vi "Upload Firmware.vi"(5 "Progress Bar":refnum<vi>, 6 "AVRDUDE Timeout (45000)":u32=45000, 7 "COM Port":refnum<visa-resource-name>="COM5", 8 "Error In":errorcluster, 9 "Firmware Index":u16(ring) items=["LINX -  Serial / USB", "LINX -  Serial / USB [Debug] "], 10 "Device Index":u16=1, 11 "Family Index":dbl=1.0) -> (0 "Error Out":errorcluster={"status"=TRUE, "code"=-1073807346, "source"="VISA Open in LVH-LINX.lvlib:Upload Firmware.vi"}, 2 "Success?":bool)   [LabVIEW 2011, in "LVH-LINX.lvlib"]
uses:
  LVH-LINX.lvlib
  Type Defs/All Firmware Data FGV States.ctl
  <vilib>/LabVIEW Hacker/LVH-Toolbox/Common/LVH-Common.lvlib
  Type Defs/Devices - Arduino.ctl
  Type Defs/Devices - Digilent.ctl
  Device/Device.lvlib
panel:
  out "Success?":bool
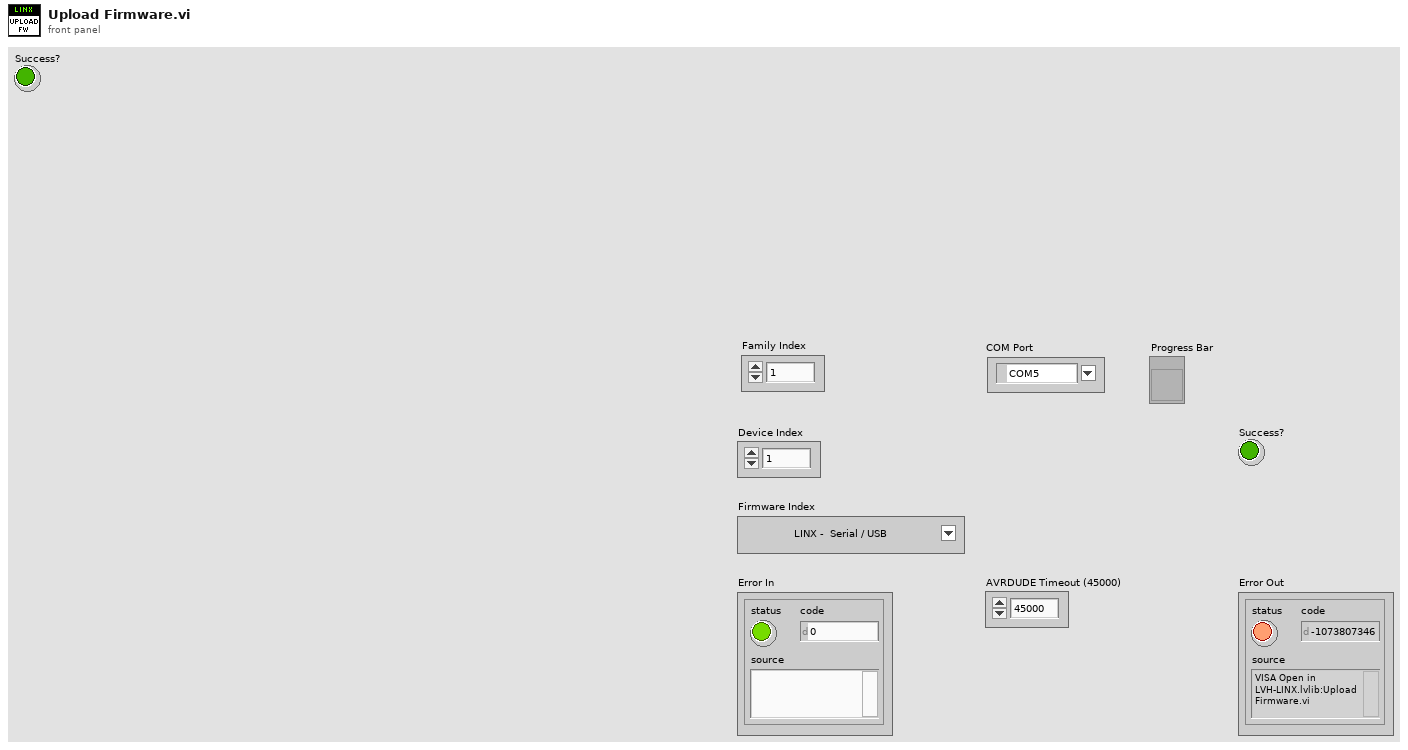
[diagram p1: front panel]
types:
  T1 = typedef "LVH-LINX.lvlib/Devices - Digilent.ctl" = enum16{"chipKIT Uno32", "chipKIT uC32", "chipKIT Max32", "chipKIT WF32"}
  T2 = typedef "LVH-LINX.lvlib/Devices - Arduino.ctl" = enum16{"Uno", "Mega 2560", "Leonardo", "Due", "Yun", "Nano", "Pro Mini", "Pro", "Fio", "Mega1280"}
  T3 = typedef "LVH-LINX.lvlib/All Firmware Data FGV States.ctl" = enum16{"Set", "Get"}
  T4 = typedef "LVH-LINX.lvlib/Generic Device.ctl" = cluster{"DI Channels":u8[], "DO Channels":u8[], "AI":u8[], "AO":u8[], "PWM":u8[], "QE":u8[], "UART":u8[], "I2C 2":u8[], "SPI":u8[], "CAN":u8[], "AI Ref (V)":dbl, "Firmware Program Interfaces":enum16{"N/A", "Serial / USB", "USB", "TCP"}[], "Firmware Versions":T5[], "Name":string, "AO Resolution (Bits)":u8, "AO Ref (V)":dbl}
  T5 = typedef "LVH-LINX.lvlib/Firmware Version.ctl" = cluster{"Name":string, "Relative Path":string, "Firmware Interface":T6}
  T6 = typedef "LVH-LINX.lvlib/Firmware Interface.ctl" = enum32{"Serial ", "Ethernet", "WIFI"}
  T7 = typedef "LVH-LINX.lvlib/Device Firmware.ctl" = cluster{"Firmware Name":string, "Firmware Path":path, "Description":string, "LINX Interface":string, "Flash Util Working Dir":path, "Flash Util Name":string, "Flash Util Args":string, "Flash Timeout (ms)":i32}
  T8 = typedef "LVH-LINX.lvlib/Device Data.ctl" = cluster{"Family ID":i32, "Family Name":string, "Device ID":i32, "Device Name":string, "Firmware Program Interfaces":string[], "Path":path}
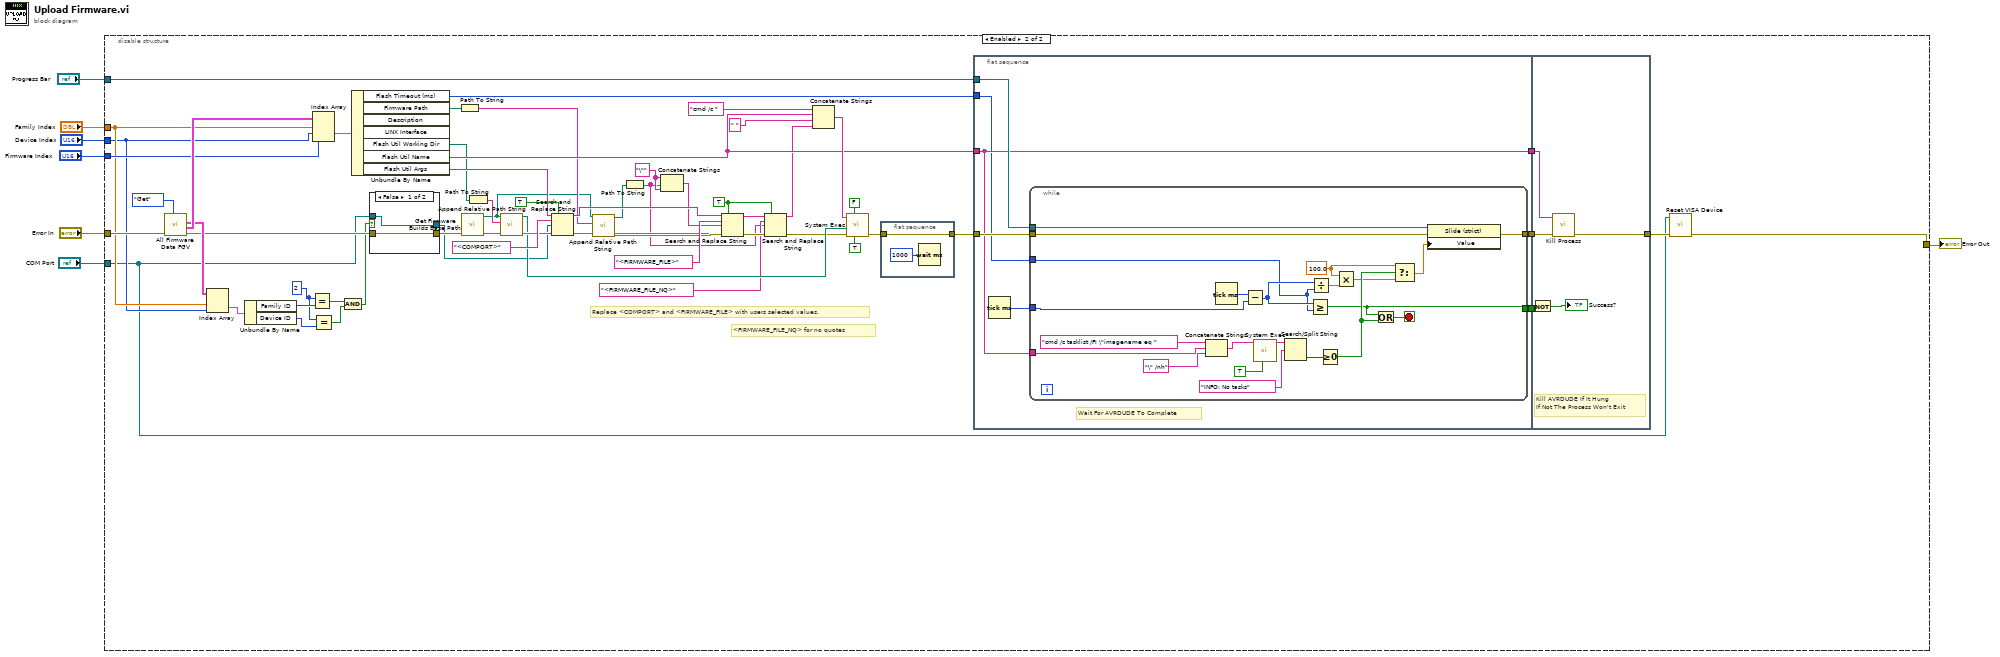
[diagram p0: block diagram]
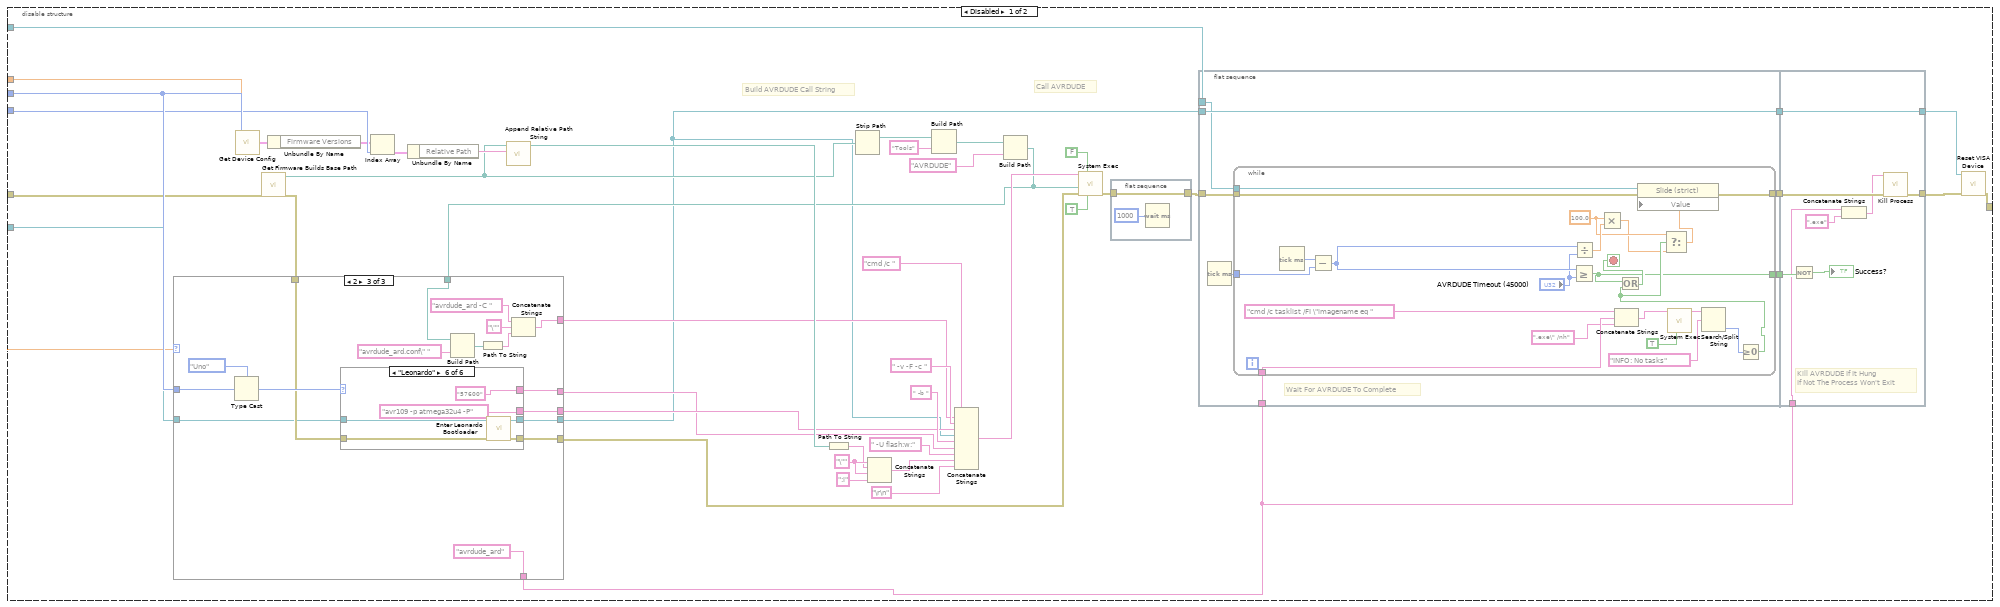
[diagram p2: hidden frame]
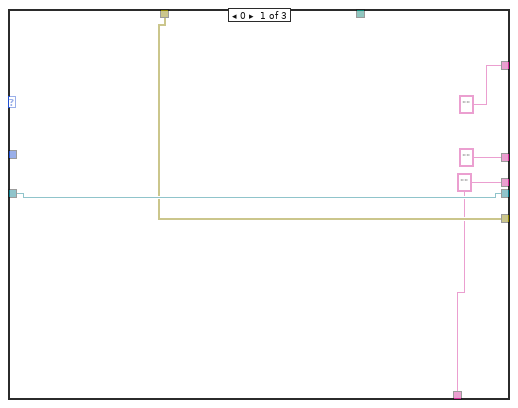
[diagram p3: hidden frame]
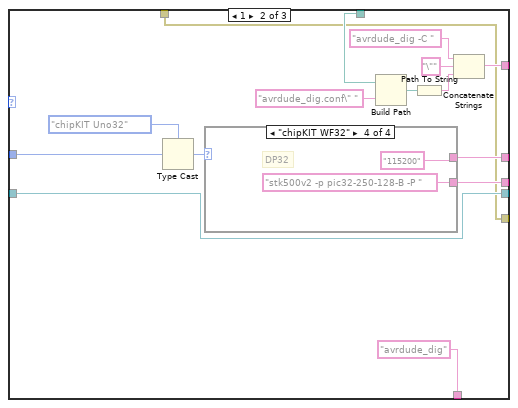
[diagram p4: hidden frame]
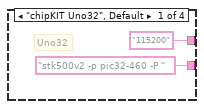
[diagram p5: hidden frame]
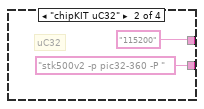
[diagram p6: hidden frame]
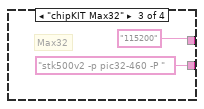
[diagram p7: hidden frame]
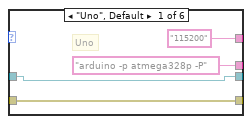
[diagram p8: hidden frame]
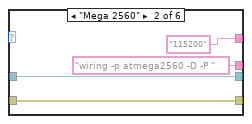
[diagram p9: hidden frame]
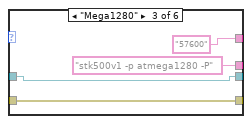
[diagram p10: hidden frame]
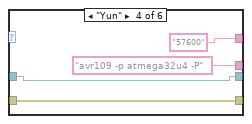
[diagram p11: hidden frame]
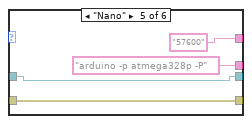
[diagram p12: hidden frame]
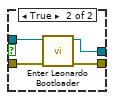
[diagram p13: hidden frame]
diagram:
  n1 = disable-structure shown="Enabled" {
    disable-tunnel: "Device Index" -> [w42 w182]
    disable-tunnel: "Family Index" -> [w38 w183]
    disable-tunnel: "Error In" -> [w31 w220]
    disable-tunnel: "Firmware Index" -> [w30 w217]
    disable-tunnel: "Progress Bar" -> [w26 w201]
    disable-tunnel: [w24 w203] -> w2
    disable-tunnel: "COM Port" -> [w12 w171]
    frame Disabled {
      w45 = "\"" ("string")
      # "Call AVRDUDE"
      # "Build AVRDUDE Call String"
      n2 = call "Get Device Config.vi"("Device ID"=w42, "Device Family"=w38) -> ("Device Config"=w28:T4)
      n3 = call "Get Firmware Builds Base Path.vi"("Error In"=w31) -> ("Error Out"=w14:errorcluster, "Firmware Builds Base Path"=w39:path)  [unwired: 9 in]
      n4 = Unbundle By Name(w28) -> ("Firmware Versions"=w29:T5[])
      n5 = Index Array(array=w29, index=w30) -> (element=w40:T5)
      n6 = Unbundle By Name(w40) -> ("Relative Path"=w41:string)
      n7 = call <vilib>:"Append Relative Path String.vi"("Relative Path"=w41, "Base Path"=w39) -> ("Absolute Path"=w43:path)  [unwired: 8 in, 1 out]
      n8 = Path To String(path=w43) -> (string=w44:string)
      n9 = Strip Path(path=w39) -> (stripped path=w32:path)  [unwired: 1 out]
      n10 = Concatenate Strings(w45, w44, w45, ":i" ("string")) -> (w21:string)
      n11 = Build Path(base path=w32, name or relative path="Tools") -> (appended path=w34:path)
      n12 = Build Path(base path=w34, name or relative path="AVRDUDE") -> (appended path=w15:path)
      n13 = case shown="2" w38 {
        tunnel: [w54 w73 w95] -> w36
        tunnel: w42 -> [_ w71 w96]
        tunnel: ["" ("string") w69 w94] -> w19
        tunnel: ["" ("string") w65 w89] -> w17
        tunnel: w15 -> [_ w68 w88]
        tunnel: w14 -> [w56 w61 w87]
        tunnel: [w56 w61 w86] -> w13
        tunnel: w12 -> [w57 w62 w85]
        tunnel: [w57 w62 w84] -> w11
        tunnel: [w54 "avrdude_dig" ("string") "avrdude_ard" ("string")] -> w8
        frame 0 {
          w54 = "" ("string")
        }
        frame 1 {
          n14 = Type Cast(type=Devices_-_Digilent."chipKIT Uno32" ("Digilent Device"), x=w71) -> (*(type *) &x=w72:T1)
          n15 = case shown="\"chipKIT WF32\"" w72 {
            tunnel: ["stk500v2 -p pic32-460 -P " ("string") "stk500v2 -p pic32-360 -P " ("string") "stk500v2 -p pic32-460 -P " ("string") "stk500v2 -p pic32-250-128-B -P " ("string")] -> w73
            tunnel: ["115200" ("string") "115200" ("string") "115200" ("string") "115200" ("string")] -> w69
            frame "chipKIT Uno32", Default {
              # "Uno32"
            }
            frame "chipKIT uC32" {
              # "uC32"
            }
            frame "chipKIT Max32" {
              # "Max32"
            }
            frame "chipKIT WF32" {
              # "DP32"
            }
          }
          n16 = Build Path(base path=w68, name or relative path="avrdude_dig.conf\" ") -> (appended path=w66:path)
          n17 = Path To String(path=w66) -> (string=w63:string)
          n18 = Concatenate Strings("avrdude_dig -C " ("string"), "\"" ("string"), w63) -> (w65:string)
        }
        frame 2 {
          n19 = Type Cast(type=Devices_-_Arduino."Uno" ("Arduino Device"), x=w96) -> (*(type *) &x=w97:T2)
          n20 = case shown="\"Leonardo\"" w97 {
            tunnel: ["arduino -p atmega328p -P" "wiring -p atmega2560 -D -P " "stk500v1 -p atmega1280 -P" "avr109 -p atmega32u4 -P" "arduino -p atmega328p -P" "avr109 -p atmega32u4 -P"] -> w95
            tunnel: ["115200" ("string") "115200" ("string") "57600" ("string") "57600" ("string") "57600" ("string") "57600" ("string")] -> w94
            tunnel: w87 -> [w99 w103 w107 w111 w115 w122]
            tunnel: [w99 w103 w107 w111 w115 w121] -> w86
            tunnel: w85 -> [w100 w104 w108 w112 w116 w120]
            tunnel: [w100 w104 w108 w112 w116 w119] -> w84
            frame "Uno", Default {
              # "Uno"
            }
            frame "Mega 2560" {
            }
            frame "Mega1280" {
            }
            frame "Yun" {
            }
            frame "Nano" {
            }
            frame "Leonardo" {
              n21 = call "Enter Leonardo Bootloader.vi"("Error In"=w122, "VISA resource name"=w120) -> ("Error Out"=w121:errorcluster, "VISA resource name"=w119:refnum<visa-resource-name>)  [unwired: 7 in, 1 out]
            }
          }
          n22 = Build Path(base path=w88, name or relative path="avrdude_ard.conf\" ") -> (appended path=w92:path)
          n23 = Path To String(path=w92) -> (string=w90:string)
          n24 = Concatenate Strings("avrdude_ard -C " ("string"), "\"" ("string"), w90) -> (w89:string)
        }
      }
      n25 = Concatenate Strings("cmd /c " ("string"), w17, " -v -F -c " ("string"), w36, w11, " -b " ("string"), w19, " -U flash:w:" ("string"), w21, "\r\n") -> (w27:string)
      n26 = call <vilib>:"System Exec.vi"("run minimized? (F)"=TRUE, "wait until completion? (T)"=FALSE, "error in (no error)"=w13, "working directory"=w15, "command line"=w27) -> ("error out"=w10:errorcluster)  [unwired: 3 in, 3 out]
      n27 = flat-sequence {
        tunnel: [w53] -> w9
        tunnel: w10 -> [w53]
        frame #0 {
          n28 = Wait (ms)(milliseconds to wait=u32 1000) -> ()  [unwired: 1 out]
        }
      }
      n29 = flat-sequence {
        tunnel: w9 -> [w128]
        tunnel: [w129] -> w51
        tunnel: [w130] -> w50
        tunnel: w11 -> [w130]
        tunnel: w26 -> [w127]
        tunnel: [w126] -> w49
        tunnel: w8 -> [w125]
        tunnel: w51 -> [w161]
        tunnel: w50 -> [w159]
        tunnel: [w160] -> w25
        tunnel: [w159] -> w23
        tunnel: w49 -> [w158]
        tunnel: w8 -> [w156]
        frame #0 {
          # "Wait For AVRDUDE To Complete"
          n30 = Tick Count (ms)() -> (millisecond timer value=w131:u32)
          n31 = while {
            tunnel: w131 -> [w152]
            tunnel: [w151] -> w129
            tunnel: w128 -> [w150]
            tunnel: w127 -> [w149]
            tunnel: [w136] -> w126
            tunnel: w125 -> [w133]
            stop <- w142 stop-if-true
            w139 = 100.0 ("x")
            n32 = Tick Count (ms)() -> (millisecond timer value=w153:u32)
            n33 = Subtract(x=w153, y=w152) -> (x-y=w148:u32)
            n34 = Greater Or Equal?(x=w148, y="AVRDUDE Timeout (45000)") -> (x >= y?=w136:bool)
            n35 = Divide(x=w148, y="AVRDUDE Timeout (45000)") -> (x/y=w146:dbl)
            n36 = Multiply(x=w139, y=w146) -> (x*y=w138:dbl)
            n37 = Concatenate Strings("cmd /c tasklist /FI \"imagename eq " ("command line"), w133, ".exe\" /nh" ("string")) -> (w134:string)
            n38 = call <vilib>:"System Exec.vi"("run minimized? (F)"=TRUE, "command line"=w134) -> ("standard output"=w144:string)  [unwired: 6 in, 3 out]
            n39 = Search/Split String(string=w144, search string/char (-)="INFO: No tasks") -> (offset of match=w141:i32)  [unwired: 1 in, 2 out]
            n40 = Greater Or Equal To 0?(x=w141) -> (x >= 0?=w140:bool)
            n41 = Or(x=w136, y=w140) -> (x .or. y?=w142:bool)
            n42 = Select(t=w139, s=w140, f=w138) -> (s? t:f=w137:dbl)
            n43 = property class="Slide (strict)"(reference=w149, error in=w150, "Value"=w137) -> (error out=w151:errorcluster)  [unwired: 1 out]
          }
        }
        frame #1 {
          # "Kill AVRDUDE If It Hung\nIf Not The Process Won't Exit"
          n44 = Not(x=w158) -> (.not. x?=→"Success?":bool)
          n45 = Concatenate Strings(w156, ".exe" ("string")) -> (w154:string)
          n46 = call <vilib>:"Kill Process.vi"("Error In"=w161, "Process Name"=w154) -> ("Error Out"=w160:errorcluster)  [unwired: 9 in]
        }
      }
      n47 = call "Reset VISA Device.vi"("Error In"=w25, "VISA resource name"=w23) -> ("Error Out"=w24:errorcluster)  [unwired: 9 in]
    }
    frame Enabled {
      w170 = "\""
      w178 = 2 ("x")
      w162 = TRUE ("replace all? (F)")
      # "<FIRMWARE_FILE_NQ> for no quotes"
      # "Replace <COMPORT> and <FIRMWARE_FILE> with users selected values."
      n48 = call "All Firmware Data FGV.vi"("All Firmware Data FGV States"=All_Firmware_Data_FGV_States."Get", "Error In"=w220) -> ("Error Out"=w174:errorcluster, "Firmwares"=w218:T7[][][], "Devices"=w184:T8[][])  [unwired: 6 in, 1 out]
      n49 = Index Array(array=w184, index (row)=w183, index (col)=w182) -> (element=w181:T8)
      n50 = Unbundle By Name(w181) -> ("Family ID"=w180:i32, "Device ID"=w179:i32)
      n51 = Equal?(x=w178, y=w180) -> (x = y?=w176:bool)
      n52 = Index Array(array=w218, index (dim 0)=w183, index (dim 1)=w182, index (dim 2)=w217) -> (element=w216:T7)
      n53 = Equal?(x=w178, y=w179) -> (x = y?=w177:bool)
      n54 = And(x=w176, y=w177) -> (x .and. y?=w173:bool)
      n55 = Unbundle By Name(w216) -> ("Flash Timeout (ms)"=w185:i32, "Firmware Path"=w196:path, "Flash Util Working Dir"=w190:path, "Flash Util Name"=w200:string, "Flash Util Args"=w210:string)  [unwired: 2 out]
      n56 = case shown="False" w173 {
        tunnel: [w221 w226] -> w175
        tunnel: w174 -> [w221 w225]
        tunnel: [w222 w224] -> w172
        tunnel: w171 -> [w222 w223]
        frame False {
        }
        frame True {
          n57 = call "Enter Leonardo Bootloader.vi"("Error In"=w225, "VISA resource name"=w223) -> ("Error Out"=w226:errorcluster, "VISA resource name"=w224:refnum<visa-resource-name>)  [unwired: 7 in, 1 out]
        }
      }
      n58 = Path To String(path=w196) -> (string=w195:string)
      n59 = call "Get Firmware Builds Base Path.vi"("Error In"=w175) -> ("Error Out"=w192:errorcluster, "Firmware Builds Base Path"=w186:path)  [unwired: 9 in]
      n60 = Path To String(path=w190) -> (string=w189:string)
      n61 = call <vilib>:"Append Relative Path String.vi"("Error In"=w192, "Relative Path"=w189, "Base Path"=w186) -> ("Error Out"=w191:errorcluster, "Absolute Path"=w188:path)  [unwired: 7 in]
      n62 = Search and Replace String(replace all?=TRUE ("replace all? (F)"), input string=w210, search string="<COMPORT>", replace string=w172, error in=w191) -> (result string=w197:string, error out=w187:errorcluster)  [unwired: 3 in, 2 out]
      n63 = call <vilib>:"Append Relative Path String.vi"("Error In"=w187, "Relative Path"=w195, "Base Path"=w186) -> ("Error Out"=w193:errorcluster, "Absolute Path"=w194:path)  [unwired: 7 in]
      n64 = Path To String(path=w194) -> (string=w165:string)
      n65 = Concatenate Strings(w170, w165, w170) -> (w169:string)
      n66 = Search and Replace String(replace all?=w162, input string=w197, search string="<FIRMWARE_FILE>", replace string=w169, error in=w193) -> (result string=w168:string, error out=w167:errorcluster)  [unwired: 3 in, 2 out]
      n67 = Search and Replace String(replace all?=w162, input string=w168, search string="<FIRMWARE_FILE_NQ>", replace string=w165, error in=w167) -> (result string=w164:string, error out=w163:errorcluster)  [unwired: 3 in, 2 out]
      n68 = Concatenate Strings("cmd /c " ("string"), w200, " " ("string"), w164) -> (w207:string)
      n69 = call <vilib>:"System Exec.vi"("run minimized? (F)"=TRUE, "wait until completion? (T)"=FALSE, "error in (no error)"=w163, "working directory"=w188, "command line"=w207) -> ("error out"=w213:errorcluster)  [unwired: 3 in, 3 out]
      n70 = flat-sequence {
        tunnel: [w262] -> w202
        tunnel: w213 -> [w262]
        frame #0 {
          n71 = Wait (ms)(milliseconds to wait=u32 1000) -> ()  [unwired: 1 out]
        }
      }
      n72 = flat-sequence {
        tunnel: w202 -> [w231]
        tunnel: [w232] -> w206
        tunnel: w201 -> [w230]
        tunnel: [w229] -> w205
        tunnel: w200 -> [w228]
        tunnel: [w228] -> w199
        tunnel: w185 -> [w227]
        tunnel: w206 -> [w260]
        tunnel: [w259] -> w204
        tunnel: w205 -> [w258]
        tunnel: w199 -> [w256]
        frame #0 {
          # "Wait For AVRDUDE To Complete"
          n73 = Tick Count (ms)() -> (millisecond timer value=w233:u32)
          n74 = while {
            tunnel: w233 -> [w254]
            tunnel: [w253] -> w232
            tunnel: w231 -> [w252]
            tunnel: w230 -> [w251]
            tunnel: [w239] -> w229
            tunnel: w228 -> [w235]
            tunnel: w227 -> [w234]
            stop <- w245 stop-if-true
            w242 = 100.0 ("x")
            n75 = Concatenate Strings("cmd /c tasklist /FI \"imagename eq " ("command line"), w235, "\" /nh" ("string")) -> (w237:string)
            n76 = Tick Count (ms)() -> (millisecond timer value=w255:u32)
            n77 = Subtract(x=w255, y=w254) -> (x-y=w250:u32)
            n78 = call <vilib>:"System Exec.vi"("run minimized? (F)"=TRUE, "command line"=w237) -> ("standard output"=w247:string)  [unwired: 6 in, 3 out]
            n79 = Search/Split String(string=w247, search string/char (-)="INFO: No tasks") -> (offset of match=w244:i32)  [unwired: 1 in, 2 out]
            n80 = Greater Or Equal?(x=w250, y=w234) -> (x >= y?=w239:bool)
            n81 = Divide(x=w250, y=w234) -> (x/y=w249:dbl)
            n82 = Greater Or Equal To 0?(x=w244) -> (x >= 0?=w243:bool)
            n83 = Multiply(x=w242, y=w249) -> (x*y=w241:dbl)
            n84 = Or(x=w239, y=w243) -> (x .or. y?=w245:bool)
            n85 = Select(t=w242, s=w243, f=w241) -> (s? t:f=w240:dbl)
            n86 = property class="Slide (strict)"(reference=w251, error in=w252, "Value"=w240) -> (error out=w253:errorcluster)  [unwired: 1 out]
          }
        }
        frame #1 {
          # "Kill AVRDUDE If It Hung\nIf Not The Process Won't Exit"
          n87 = Not(x=w258) -> (.not. x?=→"Success?":bool)
          n88 = call <vilib>:"Kill Process.vi"("Error In"=w260, "Process Name"=w256) -> ("Error Out"=w259:errorcluster)  [unwired: 9 in]
        }
      }
      n89 = call "Reset VISA Device.vi"("Error In"=w204, "VISA resource name"=w171) -> ("Error Out"=w203:errorcluster)  [unwired: 9 in]
    }
  }
  "Error Out" <- w2
